vi "lsl get desc.vi"(8 "error in (no error)":errorcluster, 11 "streaminfo":T2) -> (0 "error out":errorcluster, 3 "xml_ptr":T1)   [LabVIEW 2016, in "Lab Streaming Layer.lvlib"]
doc: "extern LIBLSL_C_API lsl_xml_ptr lsl_get_desc(lsl_streaminfo info);"
uses:
  Lab Streaming Layer.lvlib
  Custom Controls/lsl_streaminfo.ctl
  Custom Controls/lsl_xml_ptr.ctl
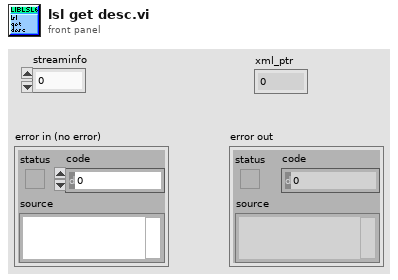
[diagram p1: front panel]
types:
  T1 = typedef "Lab Streaming Layer.lvlib/lsl_xml_ptr.ctl" = u64
  T2 = typedef "Lab Streaming Layer.lvlib/lsl_streaminfo.ctl" = u64
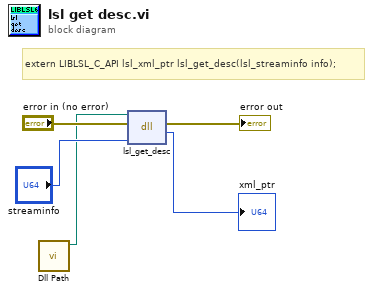
[diagram p0: block diagram]
diagram:
  # "extern LIBLSL_C_API lsl_xml_ptr lsl_get_desc(lsl_streaminfo info);"
  n1 = call "Dll Path.vi"() -> ("Dll path"=w1:path)  [unwired: 11 in]
  n2 = dll-call lib="E:/LabStreamingLayer/liblsl-LabVIEW-master/liblsl-LabVIEW-master/lsl.dll" fn="lsl_get_desc"(path in=w1, error in="error in (no error)", "info"="streaminfo") -> (error out=→"error out":errorcluster, "return type"=→"xml_ptr":u64)  [unwired: 2 in, 1 out]
